vi "SwissSPAD Live_Get All Gate Configuration Names.vi"(10 "Gate Configurations":T1[](array[typedef])) -> (2 "Gate Configuration Names":string[](array[string]))   [LabVIEW 2021]
uses:
  SwissSPAD Live_SS2 Gate Configuration.ctl
  SwissSPAD Live_SS2 Gate Definition.ctl
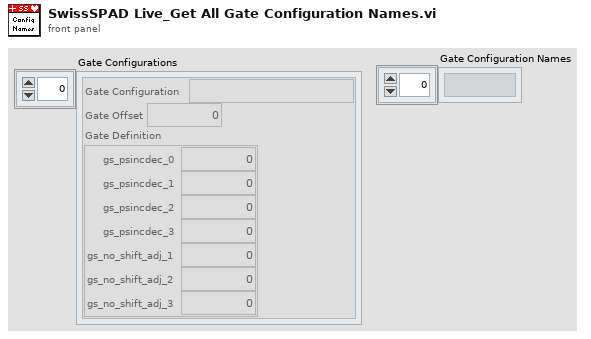
[diagram p1: front panel]
types:
  T1 = typedef "SwissSPAD Live_SS2 Gate Configuration.ctl" = cluster{"Gate Configuration":string, "Gate Offset":u32, "Gate Definition":T2}
  T2 = typedef "SwissSPAD Live_SS2 Gate Definition.ctl" = cluster{"gs_psincdec_0":u32, "gs_psincdec_1":u32, "gs_psincdec_2":u32, "gs_psincdec_3":u32, "gs_no_shift_adj_1":u32, "gs_no_shift_adj_2":u32, "gs_no_shift_adj_3":u32}
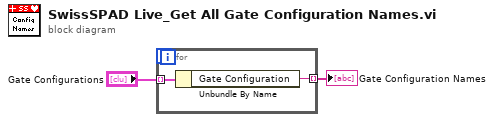
[diagram p0: block diagram]
diagram:
  n1 = for {
    tunnel: "Gate Configurations" -> [w4] mode=indexing
    tunnel: [w3] -> w1 mode=indexing
    n2 = Unbundle By Name(w4) -> ("Gate Configuration"=w3:string)
  }
  "Gate Configuration Names" <- w1
